vi "Get Selected Meas Data.vi"(0 "Build Spec":T1[](array[typedef]), 5 "Item Names":string[](array[string]), 7 "Item Symbols":i32[](array[numeric]), 11 "error in (no error)":errorcluster) -> (4 "Selected Meas":T1[](array[typedef]), 15 "error out":errorcluster)   [LabVIEW 2021, in "Packager Helpers.lvlib"]
uses:
  Packager Helpers.lvlib
  controls/Build Spec Details.ctl
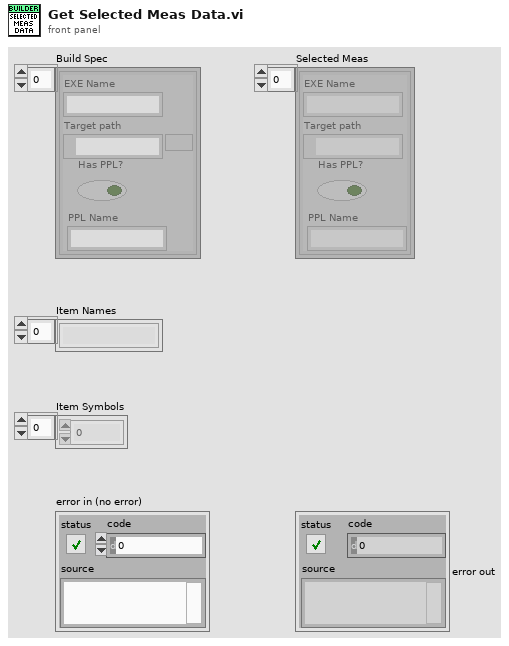
[diagram p1: front panel]
types:
  T1 = typedef "Packager Helpers.lvlib/Build Spec Details.ctl" = cluster{"EXE Name":string, "Target path":path, "Has PPL?":bool, "PPL Name":string}
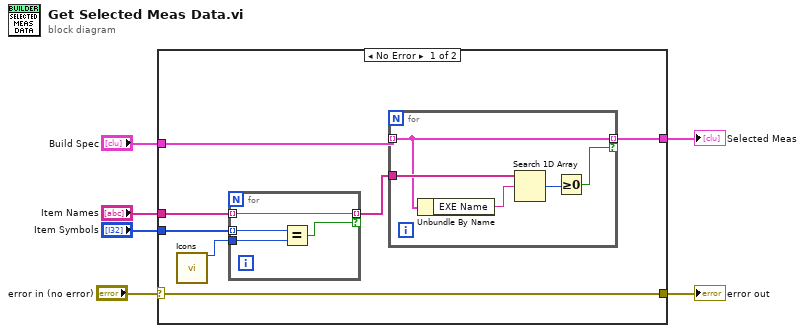
[diagram p0: block diagram]
diagram:
  n1 = case shown="No Error" "error in (no error)" {
    selector: "error in (no error)" -> [w7 w23]
    tunnel: "Item Names" -> [w12 _]
    tunnel: "Item Symbols" -> [w11 _]
    tunnel: "Build Spec" -> [w9 _]
    tunnel: [w8 _] -> w3
    tunnel: [w7 w23] -> w1
    frame No Error {
      n2 = call "Icons.vi"() -> ("Selected"=w10:i32)  [unwired: 14 in, 1 out]
      n3 = for {
        tunnel: w11 -> [w22] mode=indexing
        tunnel: w12 -> [w21] mode=indexing
        tunnel: [w21] -> w13 mode=indexing if=w20
        tunnel: w10 -> [w19]
        n4 = Equal?(x=w22, y=w19) -> (x = y?=w20:bool)
      }
      n5 = for {
        tunnel: w9 -> [w15] mode=indexing
        tunnel: w13 -> [w17]
        tunnel: [w15] -> w8 mode=indexing if=w14
        n6 = Unbundle By Name(w15) -> ("EXE Name"=w18:string)
        n7 = Search 1D Array(1D array=w17, element=w18) -> (index of element=w16:i32)  [unwired: 1 in]
        n8 = Greater Or Equal To 0?(x=w16) -> (x >= 0?=w14:bool)
      }
    }
    frame Error {
    }
  }
  "Selected Meas" <- w3
  "error out" <- w1
